vi "is Valid Ref.vi"(11 "Request in":refnum<class "Request.lvclass">) -> (2 "valid-ref?":bool)   [LabVIEW 2020, in "reqwest.lvlib" / "Request.lvclass"]
uses:
  Request.lvclass
  Request.lvclass/Request.ctl
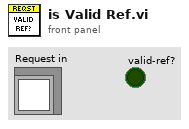
[diagram p1: front panel]
types:
  T1 = typedef "reqwest.lvlib/Request.lvclass/request_id_int.ctl" = u64
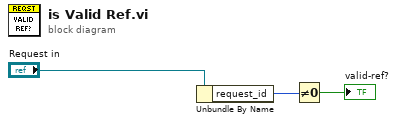
[diagram p0: block diagram]
diagram:
  n1 = Unbundle By Name("Request in") -> ("request_id"=w2:T1)
  n2 = Not Equal To 0?(x=w2) -> (x != 0?=→"valid-ref?":bool)
